vi "Teleop.vi"(10 "Match Info":T1={"Autonomous Elapsed Seconds"=0.0, "TeleOp Elapsed Seconds"=0.0, "Disabled Elapsed Seconds"=0.0, "Visited Autonomous"=FALSE, "Visited TeleOp"=FALSE, "Visited Disabled"=FALSE, "Autonomous Settings"={"Autonomous Style"=enum."Independent", "VI Refnum"=refnum}}, 11 "Call Context":T2) -> ()   [LabVIEW 2016]
doc: "This VI is called for each TeleOp packet received from the DS where the robot is not disabled. It is often used to read from the joysticks and update I/O or to update setpoints for timed control loops. It should complete and return within 20 milliseconds or it may miss DS packets."
uses:
  <vilib>/Rock Robotics/WPI/DriverStation/WPI_DriverStationDerivedRobotMode.ctl
  <vilib>/Rock Robotics/WPI/DriverStation/WPI_DriverStationMatch Info.ctl
  <vilib>/Rock Robotics/WPI/Solenoid/WPI_SolenoidValue.ctl
  Robot Global Data.vi
  <vilib>/Rock Robotics/WPI/Solenoid/WPI_SolenoidSetEnum.vi
  <vilib>/Rock Robotics/Network Tables/NT Write Number.vi
panel:
  out "IntakePistonsSelection":bool
  out "ShooterFlywVelDiv4 2":bool
  out "ShooterFlywSlaError":dbl
  out "ShooterSlaSensorVel":dbl
  out "ShooterFlywSlaEncPos":dbl
  out "ShooterFlywSlaEncVel":dbl
  out "ShooterFlywSlaCur":dbl
  out "ShooterFlywSlaThrottle":dbl
  in  "F Sla":dbl
  in  "D Sla":dbl
  in  "I Sla":dbl
  in  "P Sla":dbl
  out "ShooterFlywSlaSelection":bool
  in  "ShooterFlywSpdCmd":dbl=-0.7
  in  "IntakeMotorsCmd":dbl=0.8
  out "ConveyorSelection":bool
  in  "ConveyorCmd":dbl=-0.75
  out "ShooterUpThrottle":dbl
  out "ShooterUpEncVel":dbl
  out "ShooterUpEncPos":dbl
  out "ShooterUpCurr":dbl
  out "ShooterUptakeSelection":bool
  in  "ShooterUptakeCmd":dbl=0.75
  out "ShooterFlywVelDiv4":bool
  out "ShooterFlywError":dbl
  out "ShooterMasSensorVel":dbl
  out "ShooterFlywEncPos":dbl
  out "ShooterFlywEncVel":dbl
  out "ShooterFlywCur":dbl
  out "ShooterFlywThrottle":dbl
  in  "F Mas":dbl
  in  "D Mas":dbl
  in  "I Mas":dbl
  in  "P Mas":dbl
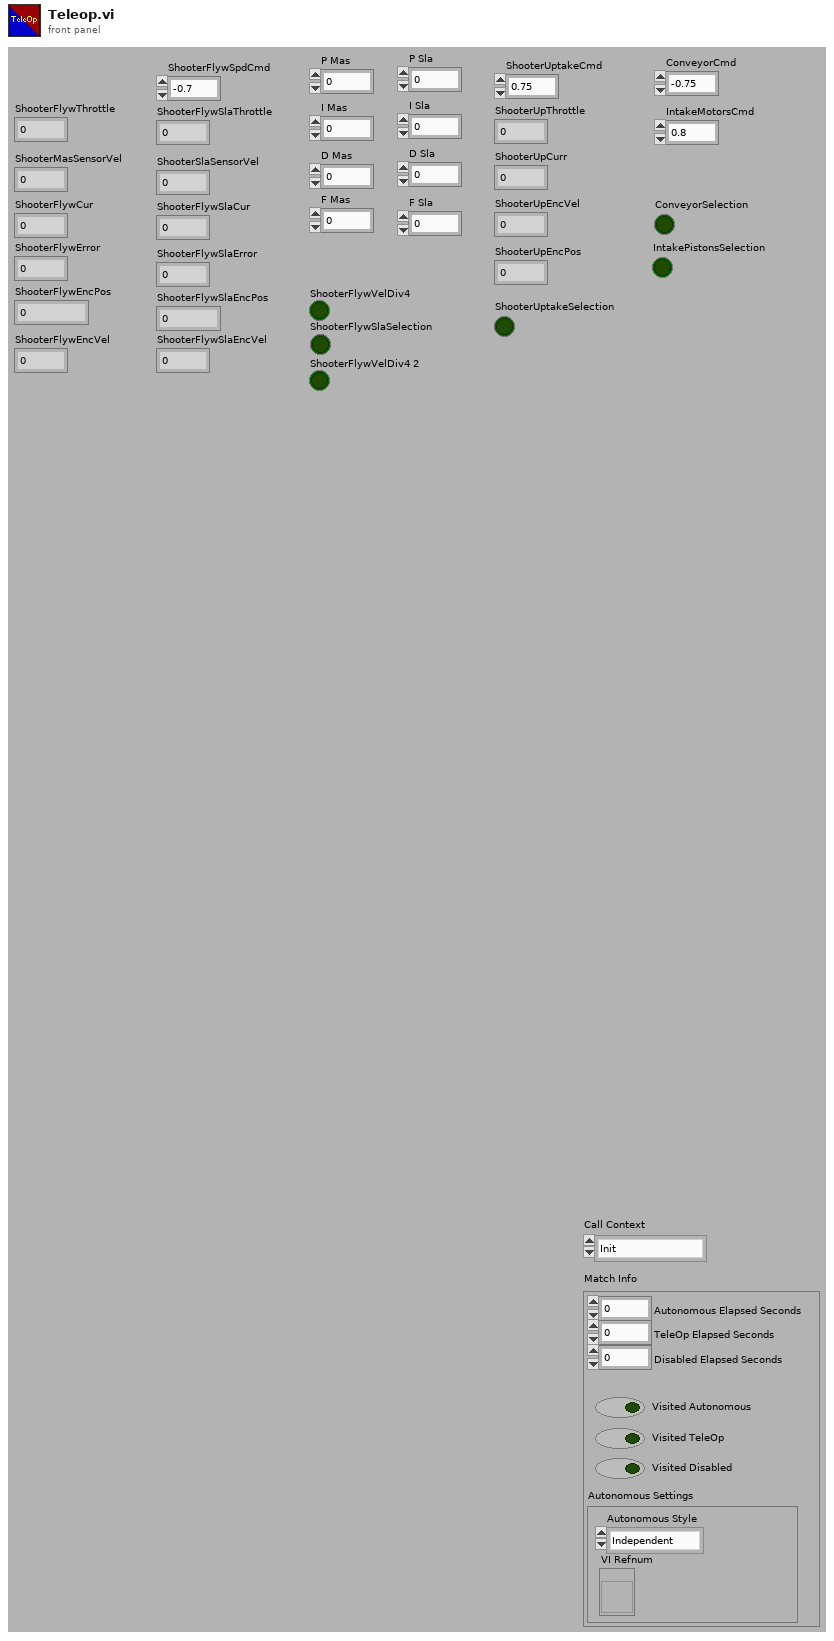
[diagram p1: front panel]
types:
  T1 = typedef "WPI_DriverStationMatch Info.ctl" = cluster{"Autonomous Elapsed Seconds":dbl, "TeleOp Elapsed Seconds":dbl, "Disabled Elapsed Seconds":dbl, "Visited Autonomous":bool, "Visited TeleOp":bool, "Visited Disabled":bool, "Autonomous Settings":cluster{"Autonomous Style":enum16{"Iterative", "Independent"}, "VI Refnum":refnum<vi>}}
  T2 = typedef "WPI_DriverStationDerivedRobotMode.ctl" = enum16{"Init", "Execute", "Stop"}
  T3 = typedef "WPI_SolenoidValue.ctl" = enum16{"Off", "On", "Forward", "Reverse"}
  T4 = typedef "WPI_MotorControlDeviceRef.ctl" = cluster{"DeviceStatus":errorcluster, "Type":T5, "PWM":cluster{"PWM Channel":T6, "DeadBand":T7}, "CAN":cluster{"Device Number":u8, "SetOutput VI Ref":variant, "GetOutput VI Ref":variant, "Enable VI Ref":variant, "Disable VI Ref":variant, "Data":variant}, "Invert":bool}
  T5 = typedef "WPI_MotorControlType.ctl" = enum16{"PWM", "CAN"}
  T6 = typedef "FPGA_DIOPWMChannel.ctl" = enum8{"PWM 0", "PWM 1", "PWM 2", "PWM 3", "PWM 4", "PWM 5", "PWM 6", "PWM 7", "PWM 8", "PWM 9", "PWM MXP 0", "PWM MXP 1", "PWM MXP 2", "PWM MXP 3", "PWM MXP 4", "PWM MXP 5", "PWM MXP 6", "PWM MXP 7", "PWM MXP 8", "PWM MXP 9", "Invalid"}
  T7 = typedef "WPI_PWMDeadband.ctl" = cluster{"Name":string, "maxPositivePwm":i32, "minPositivePwm":i32, "centerPwm":i32, "maxNegativePwm":i32, "minNegativePwm":i32, "angularRange":u16}
  T8 = typedef "WPI_SolenoidDevRef.ctl" = cluster{"DevStatus":errorcluster, "Pneumatics Control Module":u8, "Forward Solenoid Channel":T9, "Reverse Solenoid Channel":T9}
  T9 = typedef "WPI_SolenoidChannel.ctl" = enum8{"Solenoid 0", "Solenoid 1", "Solenoid 2", "Solenoid 3", "Solenoid 4", "Solenoid 5", "Solenoid 6", "Solenoid 7", "Invalid"}
  T10 = typedef "WPI_CANTalonSRX_GlobalStatus.ctl" = cluster{"Applied Throttle":dbl, "Module Enabled":bool, "CAN Error":errorcluster, "Closed Loop Error":dbl, "Forward Limit Switch Closed":bool, "Reverse Limit Switch Closed":bool, "Sensor Position":dbl, "Sensor Velocity":dbl, "Current":dbl, "Sticky Fault - Over Temp":bool, "Sticky Fault - Under Voltage":bool, "Sticky Fault - Forward Limit":bool, "Sticky Fault - Reverse Limit":bool, "Sticky Fault - Forward Soft Limit":bool, "Sticky Fault - Reverse Soft Limit":bool, "Brake is Enabled":bool, "Encoder Position":dbl, "Encoder Velocity":dbl, "Encoder Index Count":dbl, "Encoder A Pin State":bool, "Encoder B Pin State":bool, "Encoder Index Pin State":bool, "Analog In":dbl, "Analog In Velocity":dbl, "Temperature (C)":dbl, "Battery Voltage":dbl, "Control 5 Is Supported":bool, "Current Profile Slot Select":dbl, "Pos Div 8":bool, "Vel Div 4":bool, "Pulse Width Position":i32, "Pulse Width Velocity":i32, "Pulse Width Rise To Rise (us)":i32, "Pulse Width Rise To Fall (us)":i32, "Mot Prof Active Is Under Run":bool, "Mot Prof Active Has Under Run":bool, "Mot Prof Active Is Last":bool, "Mot Prof Active Velocity Only":bool, "Mot Prof Active Is Valid":bool, "Mot Prof Buffer Is Full":bool, "Mot Prof Active Profile Slot Select":i32, "Mot Prof NextID":i32, "Mot Prof Count":i32, "Mot Prof Active Velocity":dbl, "Mot Prof Active Position":dbl, "Mot Prof Output Enable":i32}
  T11 = typedef "WPI_DigitalOutputDevRef.ctl" = cluster{"DIO Channel":T12, "DevStatus":errorcluster}
  T12 = typedef "FPGA_DIOChannel.ctl" = enum8{"DIO 0", "DIO 1", "DIO 2", "DIO 3", "DIO 4", "DIO 5", "DIO 6", "DIO 7", "DIO 8", "DIO 9", "DIO MXP 0", "DIO MXP 1", "DIO MXP 2", "DIO MXP 3", "DIO MXP 4", "DIO MXP 5", "DIO MXP 6", "DIO MXP 7", "DIO MXP 8", "DIO MXP 9", "DIO MXP 10", "DIO MXP 11", "DIO MXP 12", "DIO MXP 13", "DIO MXP 14", "DIO MXP 15", "SPI Port CS1", "SPI Port CS2", "SPI Port CS3", "SPI Port MISO", "SPI Port MOSI", "Invalid"}
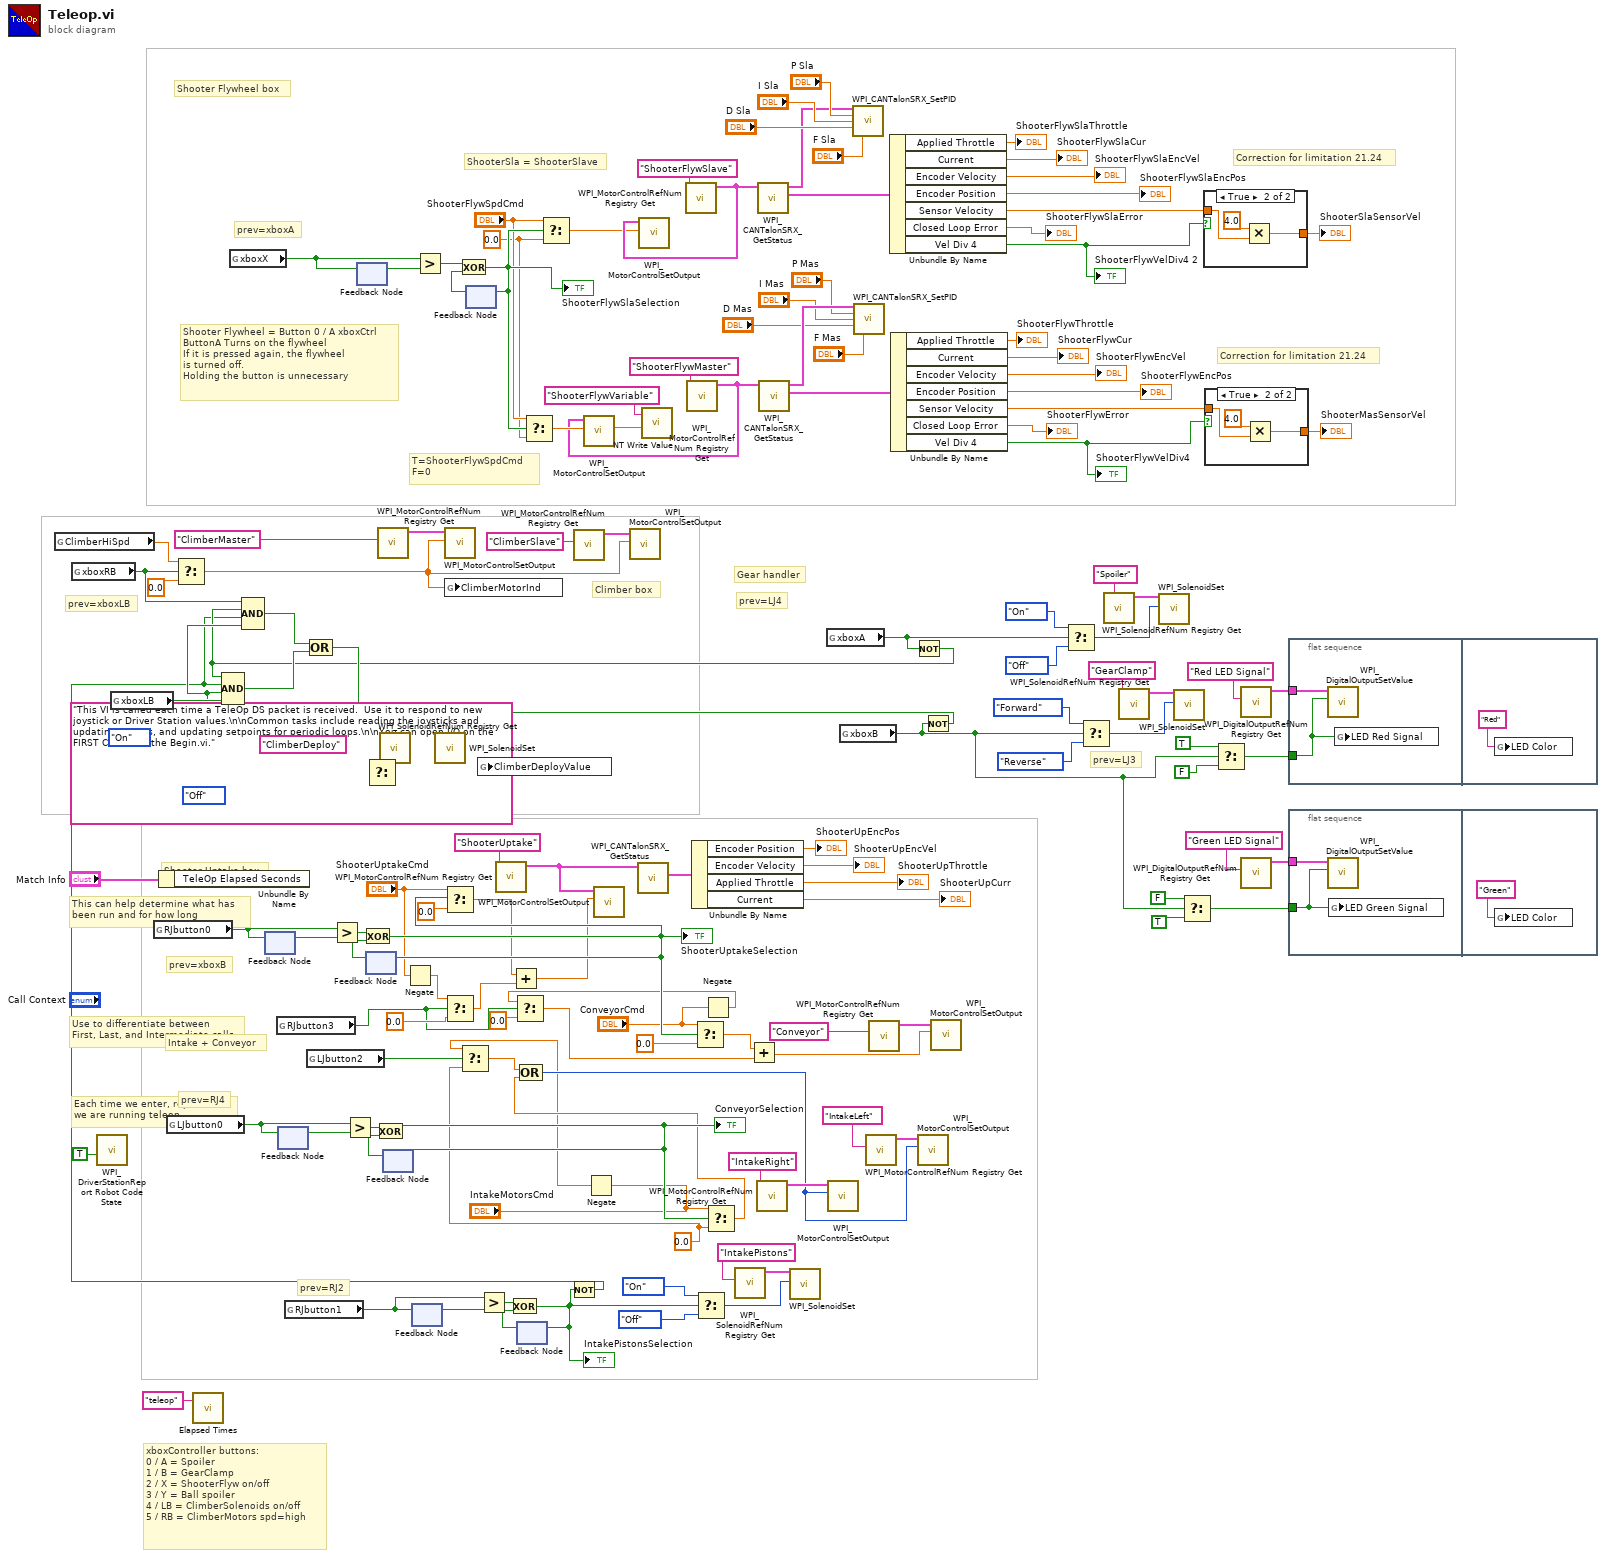
[diagram p0: block diagram]
diagram:
  w43 = 0.0 ("f")
  w37 = 0.0 ("f")
  (unwired) "This VI is called each time a TeleOp DS packet is received.  Use it to respond to new joystick or Driver Station values.\n\nCommon tasks include reading the joysticks and updating motors, and updating setpoints for periodic loops.\n\nYou can open I/O on the FIRST Call, or in the Begin.vi."
  # "T=ShooterFlywSpdCmd\nF=0"
  # "prev=LJ3"
  # "prev=LJ4"
  # "prev=xboxRB"
  # "prev=xboxLB"
  # "prev=RJ2"
  # "prev=xboxA"
  # "prev=xboxB"
  # "prev=RJ4"
  # "Gear handler"
  # "Shooter Flywheel box"
  # "ShooterSla = ShooterSlave"
  # "Correction for limitation 21.24"
  # "Intake + Conveyor"
  # "Shooter Uptake box"
  # "Climber box"
  # "Shooter Flywheel = Button 0 / A xboxCtrl\nButtonA Turns on the flywheel\nIf it is pressed again, the flywheel\nis turned off.\nHolding the button is unnecessary"
  # "xboxController buttons:\n0 / A = Spoiler\n1 / B = GearClamp\n2 / X = ShooterFlyw on/off\n3 / Y = Ball spoiler \n4 / LB = ClimberSolenoids on/off\n5 / RB = ClimberMotors spd=high"
  # "Correction for limitation 21.24"
  # "Each time we enter, report that\nwe are running teleop"
  # "Use to differentiate between\nFirst, Last, and Intermediate calls"
  # "This can help determine what has\nbeen run and for how long"
  n1 = global read "Robot Global Data.vi" "ClimberHiSpd"() -> (w100:dbl)
  n2 = global read "Robot Global Data.vi" "xboxRB"() -> (w15:bool)
  n3 = call <vilib>:"WPI_DriverStationReport Robot Code State.vi"("TeleOp"=TRUE ("Autonomous")) -> ()  [unwired: 10 in, 1 out]
  n4 = global read "Robot Global Data.vi" "xboxLB"() -> (w40:bool)
  n5 = global read "Robot Global Data.vi" "RJbutton0"() -> (w112:bool)
  n6 = Unbundle By Name("Match Info") -> ()  [unwired: 1 out]
  n7 = global read "Robot Global Data.vi" "LJbutton0"() -> (w107:bool)
  n8 = Select(t=w100, s=w15, f=0.0) -> (s? t:f=w50:dbl)
  n9 = call "Elapsed Times.vi"("Call Name"="teleop") -> ()  [unwired: 2 in, 1 out]
  n10 = global read "Robot Global Data.vi" "xboxX"() -> (w92:bool)
  n11 = feedback #1() -> (w111:bool)  [unwired: 1 in]
  n12 = feedback-in #1(w112) -> ()
  n13 = global read "Robot Global Data.vi" "RJbutton3"() -> (w20:bool)
  n14 = feedback #2() -> (w108:bool)  [unwired: 1 in]
  n15 = feedback-in #2(w107) -> ()
  n16 = global read "Robot Global Data.vi" "RJbutton1"() -> (w65:bool)
  n17 = global read "Robot Global Data.vi" "LJbutton2"() -> (w38:bool)
  n18 = Greater?(x=w112, y=w111) -> (0:w120:bool)
  n19 = Greater?(x=w107, y=w108) -> (0:w104:bool)
  n20 = feedback #3() -> (w93:bool)  [unwired: 1 in]
  n21 = feedback-in #3(w92) -> ()
  n22 = feedback #4() -> (w122:bool)  [unwired: 1 in]
  n23 = Exclusive Or(1:w122, 2:w120) -> (0:w42:bool)
  "ShooterUptakeSelection" <- w42
  n24 = feedback-in #4(w42) -> ()
  n25 = call <vilib>:"WPI_MotorControlRefNum Registry Get.vi"("refnum name"="ClimberMaster") -> ("MotorControlDevRef"=w48:T4)  [unwired: 9 in, 1 out]
  n26 = call <vilib>:"WPI_SolenoidRefNum Registry Get.vi"("refnum name"="ClimberDeploy") -> ("SolenoidDevRef"=w110:T8)  [unwired: 9 in, 1 out]
  n27 = feedback #5() -> (w103:bool)  [unwired: 1 in]
  n28 = Exclusive Or(1:w103, 2:w104) -> (0:w47:bool)
  "ConveyorSelection" <- w47
  n29 = feedback-in #5(w47) -> ()
  n30 = Negate(x="ShooterUptakeCmd") -> (-x=w26:dbl)
  n31 = feedback #6() -> (w64:bool)  [unwired: 1 in]
  n32 = feedback-in #6(w65) -> ()
  n33 = Greater?(x=w92, y=w93) -> (0:w73:bool)
  n34 = call <vilib>:"WPI_MotorControlSetOutput.vi"("Output"=w50, "MotorControlDevRef"=w48) -> ()  [unwired: 7 in, 3 out]
  n35 = global write "Robot Global Data.vi" "ClimberMotorInd"(w50) -> ()
  n36 = Select(t="ShooterUptakeCmd", s=w42, f=0.0) -> (s? t:f=w30:dbl)
  n37 = Select(t=w26, s=w20, f=0.0) -> (s? t:f=w29:dbl)
  n38 = feedback #7() -> (w75:bool)  [unwired: 1 in]
  n39 = Exclusive Or(1:w75, 2:w73) -> (0:w45:bool)
  "ShooterFlywSlaSelection" <- w45
  n40 = feedback-in #7(w45) -> ()
  n41 = Greater?(x=w65, y=w64) -> (0:w67:bool)
  n42 = call <vilib>:"WPI_MotorControlRefNum Registry Get.vi"("refnum name"="ShooterUptake") -> ("MotorControlDevRef"=w119:T4)  [unwired: 9 in, 1 out]
  n43 = Add(x=w30, y=w29) -> (x+y=w25:dbl)
  n44 = feedback #8() -> (w68:bool)  [unwired: 1 in]
  n45 = Exclusive Or(1:w68, 2:w67) -> (0:w39:bool)
  "IntakePistonsSelection" <- w39
  n46 = feedback-in #8(w39) -> ()
  n47 = Select(t="ShooterFlywSpdCmd", s=w45, f=w43) -> (s? t:f=w141:dbl)
  n48 = Select(t="ShooterFlywSpdCmd", s=w45, f=w43) -> (s? t:f=w74:dbl)
  n49 = Not(x=w39) -> (.not. x?=w1:bool)
  n50 = call <vilib>:"WPI_MotorControlRefNum Registry Get.vi"("refnum name"="ClimberSlave") -> ("MotorControlDevRef"=w95:T4)  [unwired: 9 in, 1 out]
  n51 = Negate(x="IntakeMotorsCmd") -> (-x=w33:dbl)
  n52 = Select(t=w33, s=w38, f=w37) -> (s? t:f=w36:dbl)
  n53 = call <vilib>:"WPI_MotorControlSetOutput.vi"("Output"=w25, "MotorControlDevRef"=w119) -> ()  [unwired: 7 in, 3 out]
  n54 = call <vilib>:"WPI_MotorControlSetOutput.vi"("Output"=w50, "MotorControlDevRef"=w95) -> ()  [unwired: 7 in, 3 out]
  n55 = call <vilib>:"WPI_CANTalonSRX_GetStatus.vi"("CAN Talon SRX Ref"=w119) -> ("Talon SRX Status"=w118:T10)  [unwired: 8 in, 2 out]
  n56 = call <vilib>:"WPI_MotorControlRefNum Registry Get.vi"("refnum name"="ShooterFlywSlave") -> ("MotorControlDevRef"=w76:T4)  [unwired: 9 in, 1 out]
  n57 = call <vilib>:"WPI_MotorControlSetOutput.vi"("Output"=w74, "MotorControlDevRef"=w76) -> ()  [unwired: 7 in, 3 out]
  n58 = call <vilib>:"WPI_MotorControlRefNum Registry Get.vi"("refnum name"="ShooterFlywMaster") -> ("MotorControlDevRef"=w139:T4)  [unwired: 9 in, 1 out]
  n59 = call <vilib>:"WPI_MotorControlSetOutput.vi"("Output"=w141, "MotorControlDevRef"=w139) -> ("Motor Output"=w140:dbl)  [unwired: 7 in, 2 out]
  n60 = call-poly <vilib>:"NT Write Value.vi"("Numeric"=w140, "Name"="ShooterFlywVariable") -> ()  [unwired: 9 in, 1 out]
  n61 = Unbundle By Name(w118) -> ("Encoder Position"=→"ShooterUpEncPos":dbl, "Encoder Velocity"=→"ShooterUpEncVel":dbl, "Applied Throttle"=→"ShooterUpThrottle":dbl, "Current"=→"ShooterUpCurr":dbl)
  n62 = Select(t="ConveyorCmd", s=w42, f=0.0) -> (s? t:f=w46:dbl)
  n63 = Select(t=WPI_SolenoidValue."On" ("Value"), s=w39, f=WPI_SolenoidValue."Off" ("Value")) -> (s? t:f=w66:T3)
  n64 = Negate(x="ConveyorCmd") -> (-x=w21:dbl)
  n65 = Select(t=w21, s=w20, f=0.0) -> (s? t:f=w24:dbl)
  n66 = Select(t="IntakeMotorsCmd", s=w47, f=w37) -> (s? t:f=w35:dbl)
  n67 = Compound Arithmetic op=OR(w36, w35) -> (w34:i32)
  n68 = call <vilib>:"WPI_SolenoidRefNum Registry Get.vi"("refnum name"="IntakePistons") -> ("SolenoidDevRef"=w72:T8)  [unwired: 9 in, 1 out]
  n69 = Add(x=w46, y=w24) -> (x+y=w31:dbl)
  n70 = call <vilib>:"WPI_MotorControlRefNum Registry Get.vi"("refnum name"="IntakeRight") -> ("MotorControlDevRef"=w102:T4)  [unwired: 9 in, 1 out]
  n71 = call <vilib>:"WPI_CANTalonSRX_GetStatus.vi"("CAN Talon SRX Ref"=w76) -> ("Talon SRX Status"=w83:T10, "CAN Talon SRX Ref"=w78:T4)  [unwired: 8 in, 1 out]
  n72 = call <vilib>:"WPI_CANTalonSRX_GetStatus.vi"("CAN Talon SRX Ref"=w139) -> ("Talon SRX Status"=w131:T10, "CAN Talon SRX Ref"=w136:T4)  [unwired: 8 in, 1 out]
  n73 = call-poly <vilib>:"WPI_SolenoidSet.vi"("Value"=w66, "SolenoidDevRef"=w72) -> ()  [unwired: 8 in, 2 out]
  n74 = global read "Robot Global Data.vi" "xboxA"() -> (w41:bool)
  n75 = call <vilib>:"WPI_MotorControlSetOutput.vi"("Output"=w34, "MotorControlDevRef"=w102) -> ()  [unwired: 7 in, 3 out]
  n76 = global read "Robot Global Data.vi" "xboxB"() -> (w6:bool)
  n77 = call <vilib>:"WPI_CANTalonSRX_SetPID.vi"("CAN Talon SRX Ref"=w78, "P"="P Sla", "I"="I Sla", "D"="D Sla", "F"="F Sla") -> ()  [unwired: 9 in, 2 out]
  n78 = call <vilib>:"WPI_CANTalonSRX_SetPID.vi"("CAN Talon SRX Ref"=w136, "P"="P Mas", "I"="I Mas", "D"="D Mas", "F"="F Mas") -> ()  [unwired: 9 in, 2 out]
  n79 = call <vilib>:"WPI_MotorControlRefNum Registry Get.vi"("refnum name"="IntakeLeft") -> ("MotorControlDevRef"=w63:T4)  [unwired: 9 in, 1 out]
  n80 = call <vilib>:"WPI_MotorControlRefNum Registry Get.vi"("refnum name"="Conveyor") -> ("MotorControlDevRef"=w105:T4)  [unwired: 9 in, 1 out]
  n81 = Unbundle By Name(w83) -> ("Applied Throttle"=→"ShooterFlywSlaThrottle":dbl, "Current"=→"ShooterFlywSlaCur":dbl, "Encoder Velocity"=→"ShooterFlywSlaEncVel":dbl, "Encoder Position"=→"ShooterFlywSlaEncPos":dbl, "Sensor Velocity"=w88:dbl, "Closed Loop Error"=→"ShooterFlywSlaError":dbl, "Vel Div 4"=w89:bool)
  "ShooterFlywVelDiv4 2" <- w89
  n82 = Unbundle By Name(w131) -> ("Applied Throttle"=→"ShooterFlywThrottle":dbl, "Current"=→"ShooterFlywCur":dbl, "Encoder Velocity"=→"ShooterFlywEncVel":dbl, "Encoder Position"=→"ShooterFlywEncPos":dbl, "Sensor Velocity"=w126:dbl, "Closed Loop Error"=→"ShooterFlywError":dbl, "Vel Div 4"=w125:bool)
  "ShooterFlywVelDiv4" <- w125
  n83 = Not(x=w41) -> (.not. x?=w2:bool)
  n84 = call <vilib>:"WPI_MotorControlSetOutput.vi"("Output"=w34, "MotorControlDevRef"=w63) -> ()  [unwired: 7 in, 3 out]
  n85 = Not(x=w6) -> (.not. x?=w17:bool)
  n86 = Compound Arithmetic op=AND(w2, w1, w17, w40) -> (w19:bool)
  n87 = Compound Arithmetic op=AND(w15, w2, w1, w17) -> (w16:bool)
  n88 = Compound Arithmetic op=OR(w16, w19) -> (w18:bool)
  n89 = Select(t=WPI_SolenoidValue."On" ("Value"), s=w18, f=WPI_SolenoidValue."Off" ("Value")) -> (s? t:f=w61:T3)
  n90 = call-poly <vilib>:"WPI_SolenoidSet.vi"("Value"=w61, "SolenoidDevRef"=w110) -> ()  [unwired: 8 in, 2 out]
  n91 = global write "Robot Global Data.vi" "ClimberDeployValue"(w61) -> ()
  n92 = call <vilib>:"WPI_MotorControlSetOutput.vi"("Output"=w31, "MotorControlDevRef"=w105) -> ()  [unwired: 7 in, 3 out]
  n93 = Select(t=WPI_SolenoidValue."On" ("Value"), s=w41, f=WPI_SolenoidValue."Off" ("Value")) -> (s? t:f=w55:T3)
  n94 = Select(t=WPI_SolenoidValue."Forward" ("Value"), s=w6, f=WPI_SolenoidValue."Reverse" ("Value")) -> (s? t:f=w56:T3)
  n95 = call <vilib>:"WPI_SolenoidRefNum Registry Get.vi"("refnum name"="Spoiler") -> ("SolenoidDevRef"=w54:T8)  [unwired: 9 in, 1 out]
  n96 = call <vilib>:"WPI_SolenoidRefNum Registry Get.vi"("refnum name"="GearClamp") -> ("SolenoidDevRef"=w57:T8)  [unwired: 9 in, 1 out]
  n97 = call-poly <vilib>:"WPI_SolenoidSet.vi"("Value"=w55, "SolenoidDevRef"=w54) -> ()  [unwired: 8 in, 2 out]
  n98 = call-poly <vilib>:"WPI_SolenoidSet.vi"("Value"=w56, "SolenoidDevRef"=w57) -> ()  [unwired: 8 in, 2 out]
  n99 = Select(t=FALSE, s=w6, f=TRUE) -> (s? t:f=w4:bool)
  n100 = case shown="True" w89 {
    tunnel: w88 -> [w144 w146]
    tunnel: [w144 w145] -> w90
    frame False {
    }
    frame True {
      n101 = Multiply(x=4.0, y=w146) -> (x*y=w145:dbl)
    }
  }
  "ShooterSlaSensorVel" <- w90
  n102 = case shown="True" w125 {
    tunnel: w126 -> [w148 w150]
    tunnel: [w148 w149] -> w124
    frame False {
    }
    frame True {
      n103 = Multiply(x=4.0, y=w150) -> (x*y=w149:dbl)
    }
  }
  "ShooterMasSensorVel" <- w124
  n104 = Select(t=TRUE, s=w6, f=FALSE) -> (s? t:f=w12:bool)
  n105 = call <vilib>:"WPI_DigitalOutputRefNum Registry Get.vi"("refnum name"="Red LED Signal") -> ("DigitalOutputDevRef"=w13:T11)  [unwired: 9 in, 1 out]
  n106 = call <vilib>:"WPI_DigitalOutputRefNum Registry Get.vi"("refnum name"="Green LED Signal") -> ("DigitalOutputDevRef"=w10:T11)  [unwired: 9 in, 1 out]
  n107 = flat-sequence {
    tunnel: w13 -> [w153]
    tunnel: w12 -> [w152]
    frame #0 {
      n108 = call <vilib>:"WPI_DigitalOutputSetValue.vi"("Value"=w152, "DigitalOutputDevRef"=w153) -> ()  [unwired: 8 in, 2 out]
      n109 = global write "Robot Global Data.vi" "LED Red Signal"(w152) -> ()
    }
    frame #1 {
      n110 = global write "Robot Global Data.vi" "LED Color"("Red" ("LED Color")) -> ()
    }
  }
  n111 = flat-sequence {
    tunnel: w10 -> [w156]
    tunnel: w4 -> [w155]
    frame #0 {
      n112 = call <vilib>:"WPI_DigitalOutputSetValue.vi"("Value"=w155, "DigitalOutputDevRef"=w156) -> ()  [unwired: 8 in, 2 out]
      n113 = global write "Robot Global Data.vi" "LED Green Signal"(w155) -> ()
    }
    frame #1 {
      n114 = global write "Robot Global Data.vi" "LED Color"("Green" ("LED Color")) -> ()
    }
  }
